vi "Analysis.Get List of CT Plot Image Files.vi"(11 "Data File Path":path) -> (3 "Image Files":path[](array[path]))   [LabVIEW 2024]
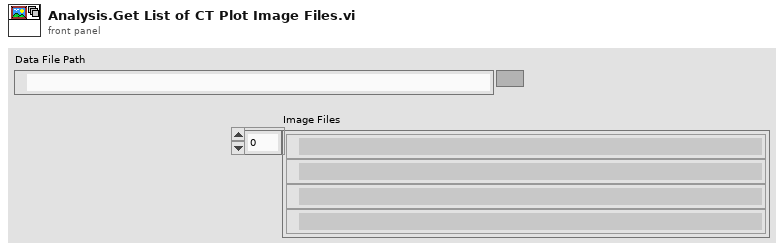
[diagram p1: front panel]
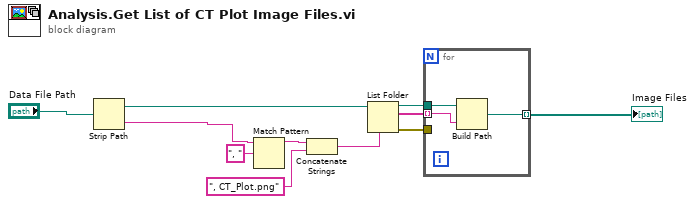
[diagram p0: block diagram]
diagram:
  n1 = Strip Path(path="Data File Path") -> (stripped path=w10:path, name=w8:string)
  n2 = Match Pattern(string=w8, regular expression=", ") -> (before substring=w5:string)  [unwired: 1 in, 3 out]
  n3 = Concatenate Strings(w5, ", CT_Plot.png") -> (w2:string)
  n4 = List Folder(path=w10, pattern=w2) -> (path out=w7:path, filenames=w6:string[], error out=w1:errorcluster)  [unwired: 2 in, 1 out]
  n5 = for {
    tunnel: w7 -> [w14]
    tunnel: w6 -> [w13] mode=indexing
    tunnel: [w12] -> w9 mode=indexing
    tunnel: w1 -> [_]
    n6 = Build Path(base path=w14, name or relative path=w13) -> (appended path=w12:path)
  }
  "Image Files" <- w9
